vi "Add_Headers.vi"(8 "error in (no error)":errorcluster, 10 "Headers":cluster{"Name":string, "Value":string}[](array[cluster]), 11 "Request in":refnum<class "Request.lvclass">) -> (0 "error out":errorcluster, 3 "Request out":refnum<class "Request.lvclass">)   [LabVIEW 2016, in "Request.lvclass"]
uses:
  Request.lvclass
  Request.lvclass/Request.ctl
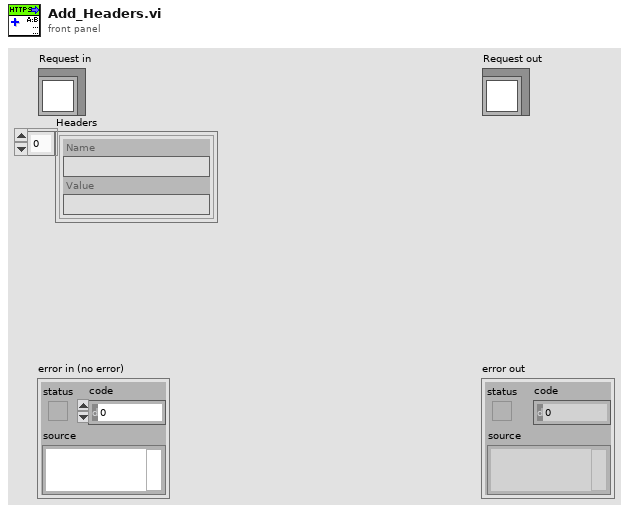
[diagram p1: front panel]
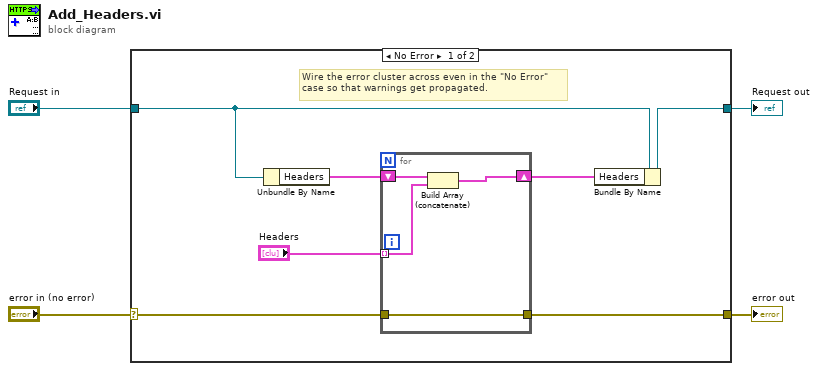
[diagram p0: block diagram]
diagram:
  n1 = case shown="No Error" "error in (no error)" {
    selector: "error in (no error)" -> [w6 w17]
    tunnel: [w5 w17] -> w3
    tunnel: [w10 w16] -> w1
    tunnel: "Request in" -> [w11 w16]
    frame No Error {
      # "Wire the error cluster across even in the \"No Error\"\ncase so that warnings get propagated."
      n2 = Unbundle By Name(w11) -> ("Headers"=w9:cluster{"Name":string, "Value":string}[])
      n3 = for {
        shift-right: [w13] -> w7
        shift-left: w9 -> [w15]
        tunnel: "Headers" -> [w14] mode=indexing
        tunnel: w6 -> [w12]
        tunnel: [w12] -> w5
        n4 = Build Array (concatenate)(w15, w14) -> (w13:cluster{"Name":string, "Value":string}[])
      }
      n5 = Bundle By Name(cluster=w11, "Headers"=w7) -> (w10:refnum<class "Request.lvclass">)
    }
    frame Error {
    }
  }
  "error out" <- w3
  "Request out" <- w1
